vi "LockStation.vi"(11 "StepName":string) -> ()   [LabVIEW 2020]
uses:
  <resource>/objmgr/ni.var.rc
panel:
  out "StationToLock":string
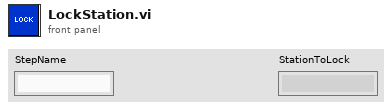
[diagram p1: front panel]
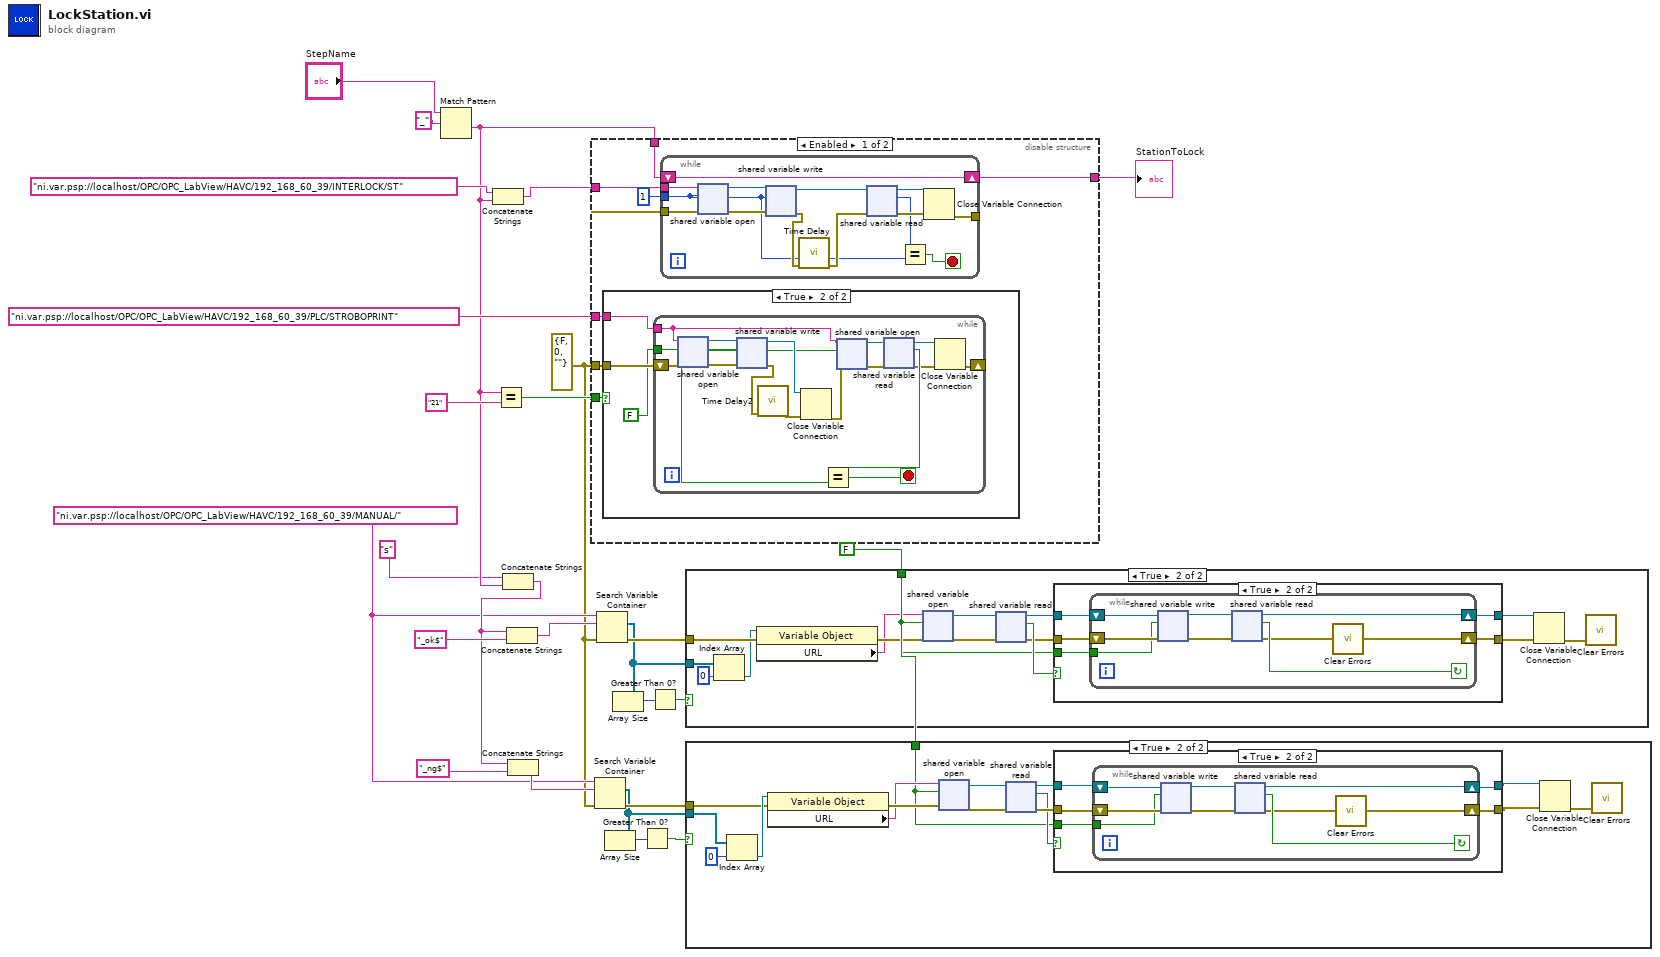
[diagram p0: block diagram]
diagram:
  w7 = FALSE
  w12 = "ni.var.psp://localhost/OPC/OPC_LabView/HAVC/192_168_60_39/MANUAL/" ("string")
  w11 = errorcluster {"status"=FALSE, "code"=0, "source"=""} ("error out")
  n1 = Match Pattern(string="StepName", regular expression="_") -> (after substring=w19:string)  [unwired: 1 in, 3 out]
  n2 = Concatenate Strings("ni.var.psp://localhost/OPC/OPC_LabView/HAVC/192_168_60_39/INTERLOCK/ST" ("string"), w19) -> (w23:string)
  n3 = Equal?(x=w19, y="21") -> (x = y?=w21:bool)
  n4 = Concatenate Strings("s", w19) -> (w14:string)
  n5 = Concatenate Strings(w14, "_ok$" ("string")) -> (w16:string)
  n6 = Concatenate Strings(w14, "_ng$" ("string")) -> (w13:string)
  n7 = disable-structure shown="Enabled" {
    disable-tunnel: w23 -> [w32 _]
    disable-tunnel: w21 -> [w31 _]
    disable-tunnel: "ni.var.psp://localhost/OPC/OPC_LabView/HAVC/192_168_60_39/PLC/STROBOPRINT" ("string") -> [w30 _]
    disable-tunnel: w19 -> [w29 w67]
    disable-tunnel: w11 -> [w28 _]
    disable-tunnel: [w27 w67] -> w10
    frame Enabled {
      n8 = case shown="True" w31 {
        tunnel: w28 -> [_ w36]
        tunnel: w30 -> [_ w34]
        frame False {
        }
        frame True {
          n9 = while {
            tunnel: w34 -> [w39]
            tunnel: FALSE -> [w37]
            shift-right: [w49] -> _
            shift-left: w36 -> [w46]
            stop <- w51 stop-if-true
            n10 = shared-variable-open(w39, w46, w37) -> (w44:refnum<k21>, w45:errorcluster)  [unwired: 1 in]
            n11 = shared-variable-write(w44, w45, w37) -> (w42:refnum<k21>, w52:errorcluster)
            n12 = call "Time Delay2"("error in (no error)"=w52) -> ("error out"=w43:errorcluster)  [unwired: 10 in]
            n13 = Close Variable Connection(8:w43, 11:w42) -> (0:w41:errorcluster)
            n14 = shared-variable-open(w39, w41, w37) -> (w38:refnum<k21>, w40:errorcluster)  [unwired: 1 in]
            n15 = shared-variable-read(w38, w40) -> (w47:refnum<k21>, w48:errorcluster, w50:bool)  [unwired: 1 out]
            n16 = Equal?(x=w50, y=w37) -> (x = y?=w51:bool)
            n17 = Close Variable Connection(8:w48, 11:w47) -> (0:w49:errorcluster)
          }
        }
      }
      n18 = while {
        tunnel: 1 -> [w56]
        tunnel: w32 -> [w64]
        shift-right: [w55] -> w27
        shift-left: w29 -> [w55]
        tunnel: [w54] -> _
        tunnel: w28 -> [w53]
        stop <- w58 stop-if-true
        n19 = shared-variable-open(w64, w53, w56) -> (w65:refnum<k21>, w66:errorcluster)  [unwired: 1 in]
        n20 = shared-variable-write(w65, w66, w56) -> (w62:refnum<k21>, w63:errorcluster)
        n21 = call "Time Delay"("error in (no error)"=w63) -> ("error out"=w61:errorcluster)  [unwired: 10 in]
        n22 = shared-variable-read(w62, w61) -> (w59:refnum<k21>, w60:errorcluster, w57:i32)  [unwired: 1 out]
        n23 = Equal?(x=w57, y=w56) -> (x = y?=w58:bool)
        n24 = Close Variable Connection(8:w60, 11:w59) -> (0:w54:errorcluster)
      }
    }
    frame Disabled {
    }
  }
  "StationToLock" <- w10
  n25 = Search Variable Container(8:w11, 10:w13, 11:w12) -> (0:w8:errorcluster, 2:w2:refnum<k21>[])  [unwired: 3 in, 1 out]
  n26 = Search Variable Container(8:w11, 10:w16, 11:w12) -> (0:w9:errorcluster, 2:w6:refnum<k21>[])  [unwired: 3 in, 1 out]
  n27 = Array Size(array=w2) -> (size(s)=w3:i32)
  n28 = Array Size(array=w6) -> (size(s)=w4:i32)
  n29 = Greater Than 0?(x=w3) -> (x > 0?=w1:bool)
  n30 = Greater Than 0?(x=w4) -> (x > 0?=w5:bool)
  n31 = case shown="True" w5 {
    tunnel: w6 -> [_ w82]
    tunnel: w9 -> [_ w80]
    tunnel: w7 -> [_ w68]
    frame False {
    }
    frame True {
      n32 = Index Array(array=w82, index=0) -> (element=w77:refnum<k21>)
      n33 = property class="Variable Object"(reference=w77, error in=w80) -> (error out=w79:errorcluster, "URL"=w78:string)  [unwired: 1 out]
      n34 = shared-variable-open(w78, w79, w68) -> (w75:refnum<k21>, w76:errorcluster)  [unwired: 1 in]
      n35 = shared-variable-read(w75, w76) -> (w72:refnum<k21>, w73:errorcluster, w74:bool)  [unwired: 1 out]
      n36 = case shown="True" w74 {
        tunnel: w73 -> [w83 w89]
        tunnel: w72 -> [w84 w88]
        tunnel: [w84 w86] -> w70
        tunnel: [w83 w87] -> w71
        tunnel: w68 -> [_ w85]
        frame False {
        }
        frame True {
          n37 = while {
            shift-right: [w91] -> w87
            shift-left: w89 -> [w98]
            shift-right: [w92] -> w86
            shift-left: w88 -> [w97]
            tunnel: w85 -> [w90]
            stop <- w94 continue-if-true
            n38 = shared-variable-write(w97, w98, w90) -> (w95:refnum<k21>, w96:errorcluster)
            n39 = shared-variable-read(w95, w96) -> (w92:refnum<k21>, w93:errorcluster, w94:bool)  [unwired: 1 out]
            n40 = call <vilib>:"Clear Errors.vi"("error in (no error)"=w93) -> ("error out"=w91:errorcluster)  [unwired: 5 in, 1 out]
          }
        }
      }
      n41 = Close Variable Connection(8:w71, 11:w70) -> (0:w69:errorcluster)
      n42 = call <vilib>:"Clear Errors.vi"("error in (no error)"=w69) -> ()  [unwired: 5 in, 2 out]
    }
  }
  n43 = case shown="True" w1 {
    tunnel: w8 -> [_ w111]
    tunnel: w7 -> [_ w99]
    tunnel: w2 -> [_ w109]
    frame False {
    }
    frame True {
      n44 = Index Array(array=w109, index=0) -> (element=w112:refnum<k21>)
      n45 = property class="Variable Object"(reference=w112, error in=w111) -> (error out=w110:errorcluster, "URL"=w106:string)  [unwired: 1 out]
      n46 = shared-variable-open(w106, w110, w99) -> (w107:refnum<k21>, w108:errorcluster)  [unwired: 1 in]
      n47 = shared-variable-read(w107, w108) -> (w104:refnum<k21>, w105:errorcluster, w103:bool)  [unwired: 1 out]
      n48 = case shown="True" w103 {
        tunnel: w105 -> [w114 w120]
        tunnel: w104 -> [w115 w119]
        tunnel: [w115 w117] -> w100
        tunnel: [w114 w118] -> w101
        tunnel: w99 -> [_ w116]
        frame False {
        }
        frame True {
          n49 = while {
            shift-right: [w122] -> w118
            shift-left: w120 -> [w129]
            shift-right: [w123] -> w117
            shift-left: w119 -> [w128]
            tunnel: w116 -> [w121]
            stop <- w125 continue-if-true
            n50 = shared-variable-write(w128, w129, w121) -> (w126:refnum<k21>, w127:errorcluster)
            n51 = shared-variable-read(w126, w127) -> (w123:refnum<k21>, w124:errorcluster, w125:bool)  [unwired: 1 out]
            n52 = call <vilib>:"Clear Errors.vi"("error in (no error)"=w124) -> ("error out"=w122:errorcluster)  [unwired: 5 in, 1 out]
          }
        }
      }
      n53 = Close Variable Connection(8:w101, 11:w100) -> (0:w102:errorcluster)
      n54 = call <vilib>:"Clear Errors.vi"("error in (no error)"=w102) -> ()  [unwired: 5 in, 2 out]
    }
  }
